vi "image2data_3d.vi"(10 "image_1d":sgl[](array[numeric]), 11 "Data":T1 {"slice orientation" items=["transverse unflipped", "coronal unflipped", "sagittal unflipped", "transverse flipped", "coronal flipped", "sagittal flipped"]}) -> (2 "imag3_3d":sgl[][][](array[numeric]), 3 "Data":T1 {"slice orientation" items=["transverse unflipped", "coronal unflipped", "sagittal unflipped", "transverse flipped", "coronal flipped", "sagittal flipped"]})   [LabVIEW 2014]
uses:
  control/head_data.ctl
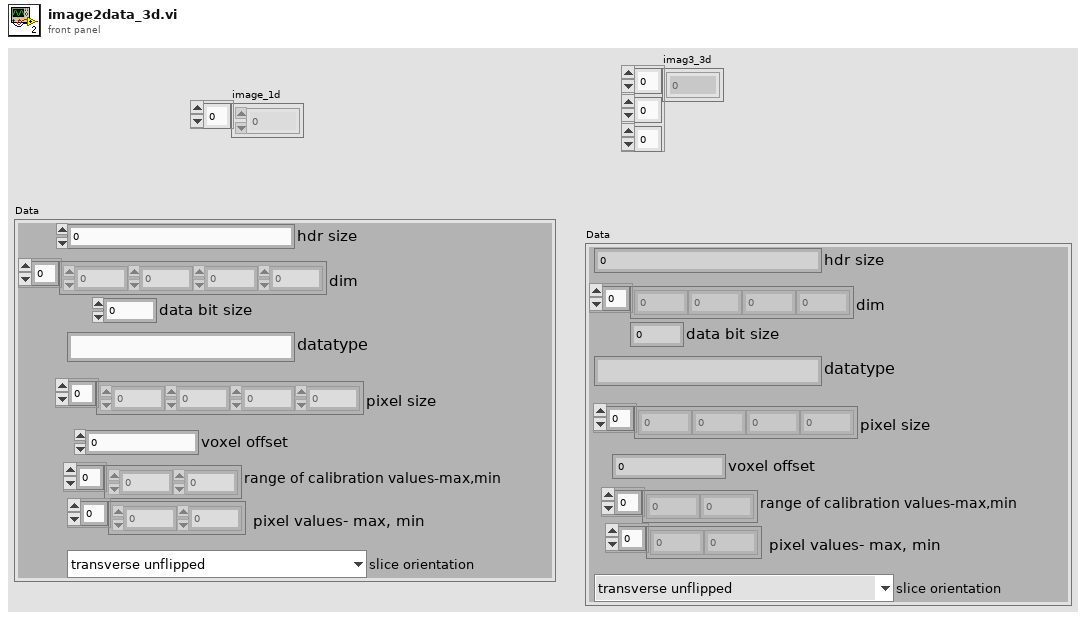
[diagram p1: front panel]
types:
  T1 = typedef "head_data.ctl" = cluster{"hdr size":i32, "dim":i32[], "data bit size":i32, "datatype":string, "pixel size ":sgl[], "voxel offset":sgl, "range of calibration values-max,min":sgl[], " pixel values- max, min":sgl[], "slice orientation":u16}
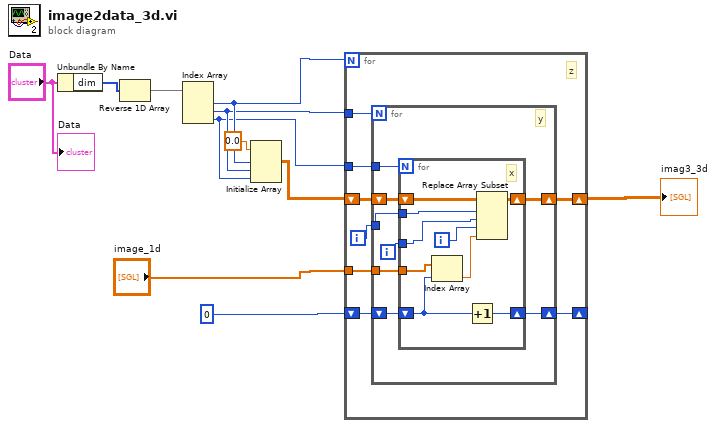
[diagram p0: block diagram]
diagram:
  n1 = Unbundle By Name("Data") -> ("dim"=w2:i32[])
  n2 = Reverse 1D Array(array=w2) -> (reversed array=w1:i32[])
  n3 = Index Array(array=w1) -> (element #1=w8:i32, element #2=w7:i32, element #3=w6:i32)  [unwired: 3 in]
  n4 = Initialize Array(sgl 0.0 ("element"), w8, w7, w6) -> (w4:sgl[][][])
  n5 = for {
    N: w8 -> [_]
    tunnel: "image_1d" -> [w19]
    shift-right: [w18] -> _
    shift-left: 0 -> [w17]
    tunnel: w6 -> [w16]
    tunnel: w7 -> [w15]
    shift-right: [w13] -> w3
    shift-left: w4 -> [w14]
    i -> [w12]
    # "z"
    n6 = for {
      N: w15 -> [_]
      tunnel: w19 -> [w27]
      shift-right: [w26] -> w18
      shift-left: w17 -> [w25]
      tunnel: w16 -> [w24]
      shift-right: [w22] -> w13
      shift-left: w14 -> [w23]
      tunnel: w12 -> [w20]
      i -> [w21]
      # "y"
      n7 = for {
        N: w24 -> [_]
        tunnel: w27 -> [w36]
        shift-right: [w35] -> w26
        shift-left: w25 -> [w34]
        shift-right: [w32] -> w22
        shift-left: w23 -> [w33]
        tunnel: w21 -> [w29]
        tunnel: w20 -> [w30]
        i -> [w28]
        # "x"
        n8 = Index Array(array=w36, index=w34) -> (element=w31:sgl)
        n9 = Increment(x=w34) -> (x+1=w35:i32)
        n10 = Replace Array Subset(array=w33, new element=w31, index (dim 0)=w30, index (dim 1)=w29, index (dim 2)=w28) -> (w32:sgl[][][])
      }
    }
  }
  "imag3_3d" <- w3
  "Data" <- "Data"
